vi "nav2.vi"(9 "Drone":T3, 11 "Field":T1[][](array[typedef])) -> (2 "Move?":bool, 3 "direction":T2 items=["^", "^>", ">", "V>", "V", "<V", "<", "<^"])   [LabVIEW 2009]
uses:
  Drone data.ctl
  direction.ctl
  square.ctl
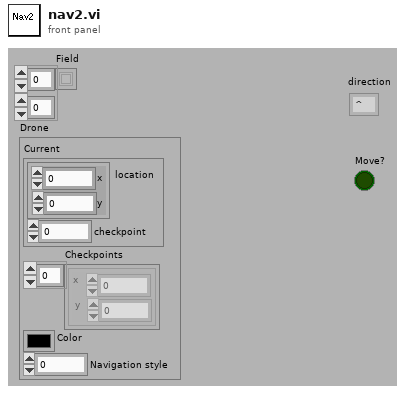
[diagram p1: front panel]
types:
  T1 = typedef "square.ctl" = u8
  T2 = typedef "direction.ctl" = i8
  T3 = typedef "Drone data.ctl" = cluster{"Current":cluster{"location":cluster{"x":i16, "y":i16}, "checkpoint":i32}, "Checkpoints":cluster{"x":i16, "y":i16}[], "Color":u32, "Navigation style":i32}
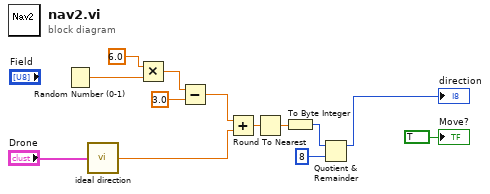
[diagram p0: block diagram]
diagram:
  n1 = Random Number (0-1)() -> (number: 0 to 1=w12:dbl)
  n2 = call "ideal direction.vi"("Drone"="Drone") -> ("ideal direction"=w7:dbl)
  n3 = Multiply(x=6.0, y=w12) -> (x*y=w10:dbl)
  n4 = Subtract(x=w10, y=3.0) -> (x-y=w8:dbl)
  n5 = Add(x=w8, y=w7) -> (x+y=w6:dbl)
  n6 = Round To Nearest(number=w6) -> (nearest integer value=w5:dbl)
  n7 = To Byte Integer(number=w5) -> (8bit integer=w4:i8)
  n8 = Quotient & Remainder(x=w4, y=i8 8) -> (x-y*floor(x/y)=→"direction":i8)  [unwired: 1 out]
  "Move?" <- TRUE ("Move?")
